vi "EOL Check Current Data.vi"(0 "Motor Type":T1, 5 "Motion Data":sgl[][](array[numeric]), 7 "Decibel data":dbl[](array[numeric]), 9 "Current Motion":T2=enum."Glass Slide Open", 11 "Audit Motion Data Cluster":T3={"Power Supply Voltage"=0.0, "Min Avg Current"=0.0, "Max Avg Current"=0.0, "Min Run Time"=0.0, "Max Run Time"=0.0, "Min Speed"=0.0, "Max Speed"=0.0, "AP Data % of Threshold"=0.0, "Travel Distance"=0.0, "AP Data Type"=enum."91/61", "Check Current"=FALSE, "Check Run Time"=FALSE, "Check Speed"=FALSE, "Express Motion?"=FALSE, "Check Sound Test"=FALSE, "Check Position?"=FALSE, "Collect AP Data"=FALSE, "Inital Position"=0, "End Position"=0, "Goto Posiition"=0, "Max max Current"=0.0, "Min max Current"=0.0, "Check max Current"=FALSE, "Check Sound"=FALSE, "Min Sound (dB)"=0.0, "Max Sound (dB)"=0.0, "SW Mode"=enum."Hard Switch", "LIN Msg"={"ID"=0, "Msg"=[], "LDF"="EX1H"}} {"LIN Msg"."Msg" format="%02x"; "LIN Msg"."ID" format="%02x"}, 12 "Error Table In":string[][](array[string])) -> (1 "max Current":dbl, 3 "Current Out":sgl[](graph), 4 "Pass? Out":bool, 6 "Run Time":dbl, 8 "Sound (dB)":dbl, 10 "Avg Current":dbl, 14 "Error Table Out":string[][](array[string]), 15 "Speed":dbl)   [LabVIEW 2018]
uses:
  05.UserVI's/type defs/17x Audit Motion Data Seq Control.ctl
  05.UserVI's/type defs/17x AP Data Type.ctl
  02.Type Def's/All Motions.ctl
  05.UserVI's/type defs/EOL Motor Type.ctl
  <vilib>/Analysis/baseanly.llb/Mean (DBL).vi
  <vilib>/Analysis/NI_AALBase.lvlib
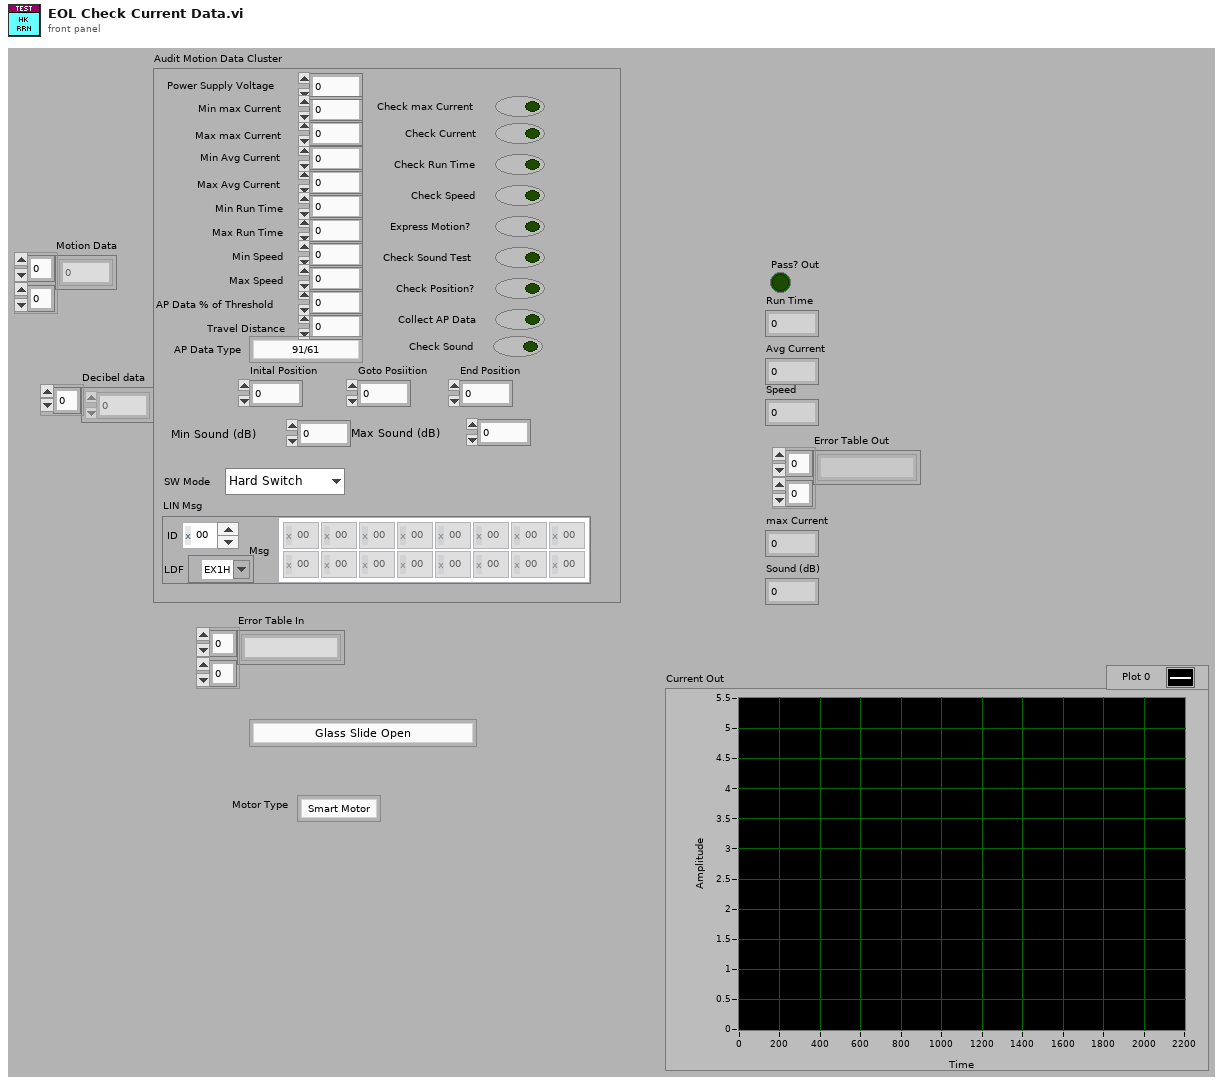
[diagram p1: front panel]
types:
  T1 = typedef "EOL Motor Type.ctl" = enum16{"Smart Motor", "Sensor Motor"}
  T2 = typedef "All Motions.ctl" = enum16{"Glass Teach", "Glass Slide Open", "Glass Slide Close", "Glass Vent Open", "Glass Vent Close", "Sunshade Teach", "Sunshade Open", "Sunshade Close", "Idle", "Sunshade Open 2", "Sunshade Close 2", "Glass Slide Open Sunshade Open", "Glass Slide Open Sunshade Close", "Glass Slide Close Sunshade Open", "Glass Slide Close Sunshade Close", "Glass Vent Open Sunshade Open", "Glass Vent Open Sunshade Close", "Glass Vent Close Sunshade Open", "Glass Vent Close Sunshade Close", "Express Glass Slide Open", "Express Glass Slide Close", "Express Glass Vent Open", "Express Glass Vent Close", "Express Sunshade Open", "Express Sunshade Close", "Express Sunshade Open 2", "Express Sunshade Close 2", "Express Glass Slide Open Sunshade Open", "Express Glass Slide Open Sunshade Close", "Express Glass Slide Close Sunshade Open", "Express Glass Slide Close Sunshade Close", "Express Glass Vent Open Sunshade Open", "Express Glass Vent Open Sunshade Close", "Express Glass Vent Close Sunshade Open", "Express Glass Vent Close Sunshade Close", "Goto Position Glass", "Goto Position Sunshade", "Sunshade Teach 2"}
  T3 = typedef "17x Audit Motion Data Seq Control.ctl" = cluster{"Power Supply Voltage":dbl, "Min Avg Current":dbl, "Max Avg Current":dbl, "Min Run Time":dbl, "Max Run Time":dbl, "Min Speed":dbl, "Max Speed":dbl, "AP Data % of Threshold":dbl, "Travel Distance":dbl, "AP Data Type":T4, "Check Current":bool, "Check Run Time":bool, "Check Speed":bool, "Express Motion?":bool, "Check Sound Test":bool, "Check Position?":bool, "Collect AP Data":bool, "Inital Position":u16, "End Position":u16, "Goto Posiition":u16, "Max max Current":dbl, "Min max Current":dbl, "Check max Current":bool, "Check Sound":bool, "Min Sound (dB)":dbl, "Max Sound (dB)":dbl, "SW Mode":enum16{"Hard Switch", "Uncond Frame"}, "LIN Msg":cluster{"ID":u8, "Msg":u8[][], "LDF":refnum<k21>}}
  T4 = typedef "17x AP Data Type.ctl" = enum16{"91/61", "92/62", "93/63", "67", "68", "6F", "71", "91 Msg", "92 Msg", "93 Msg", "94 Msg", "HiRain 91", "HiRain 92 Speed", "HiRain 92 HS", "HiRain 92", "HiRain 93", "SnT"}
  T5 = cluster{"Run Time":dbl, "Avg Current":dbl, "Speed":dbl, "Audit Motion Data Cluster":T3, "Error Table In":string[][], "Pass?":bool, "Current Motion":T2, "Motor Type":T1, "max Current":dbl, "Sound (dB)":dbl, "Decibel data":dbl[]}
  T6 = typedef "EOL Analog Input Control.ctl" = enum16{"SW PS  Volage", "Switch A", "Switch B", "Switch C", "Motor Voltage", "Motor Current", "ATS"}
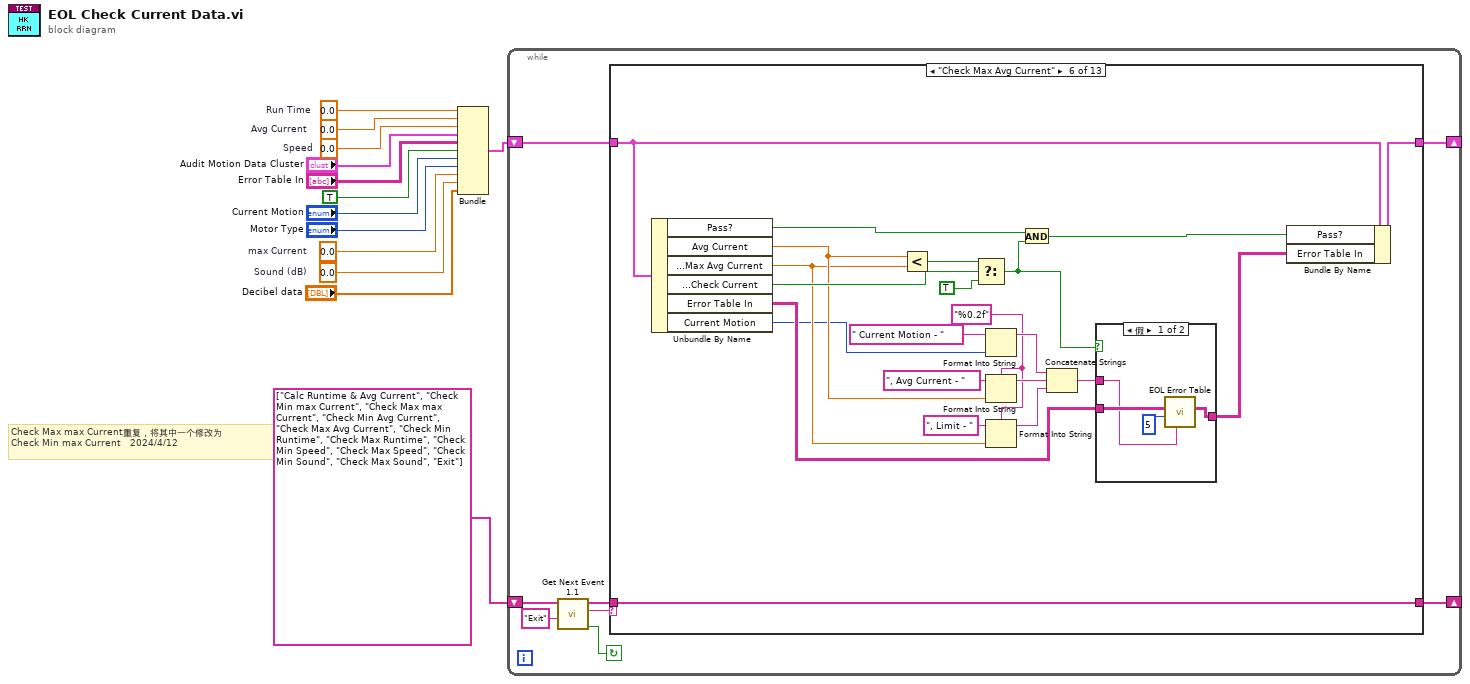
[diagram p0: block diagram]
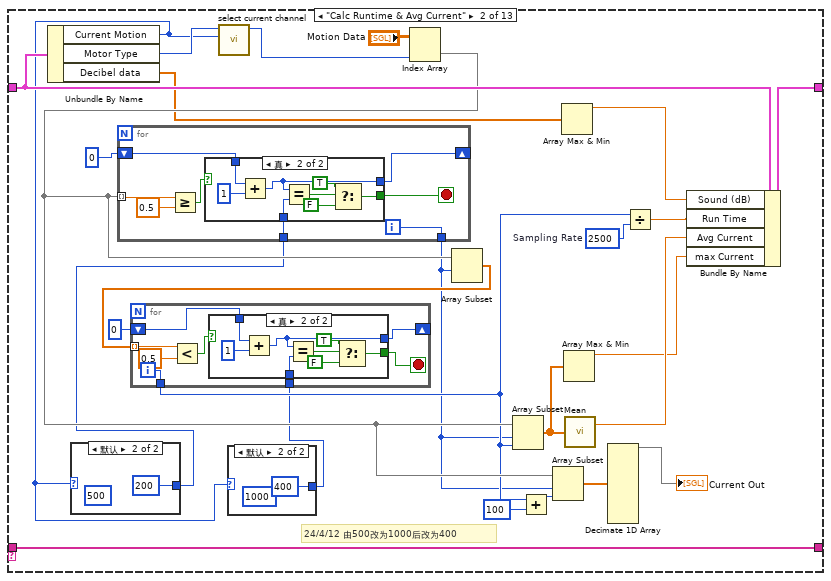
[diagram p3: hidden frame]
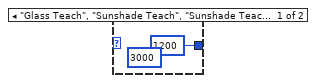
[diagram p4: hidden frame]
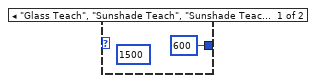
[diagram p5: hidden frame]
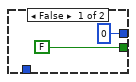
[diagram p6: hidden frame]
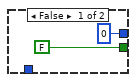
[diagram p7: hidden frame]
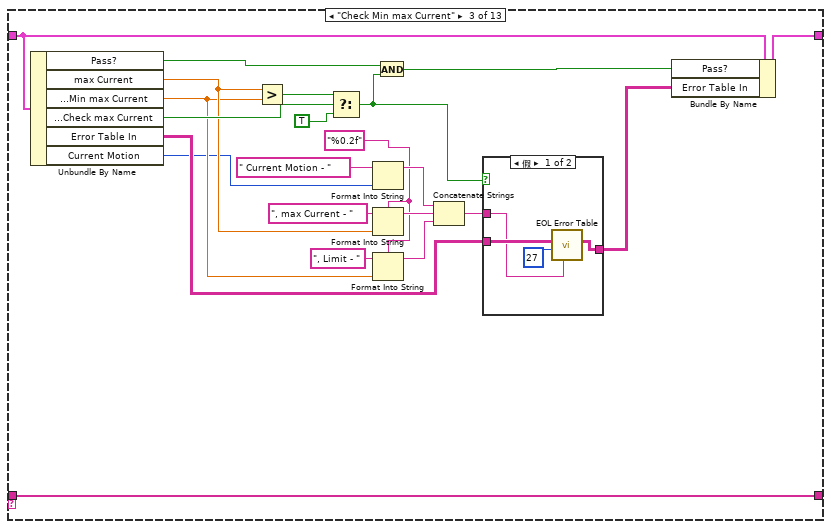
[diagram p8: hidden frame]
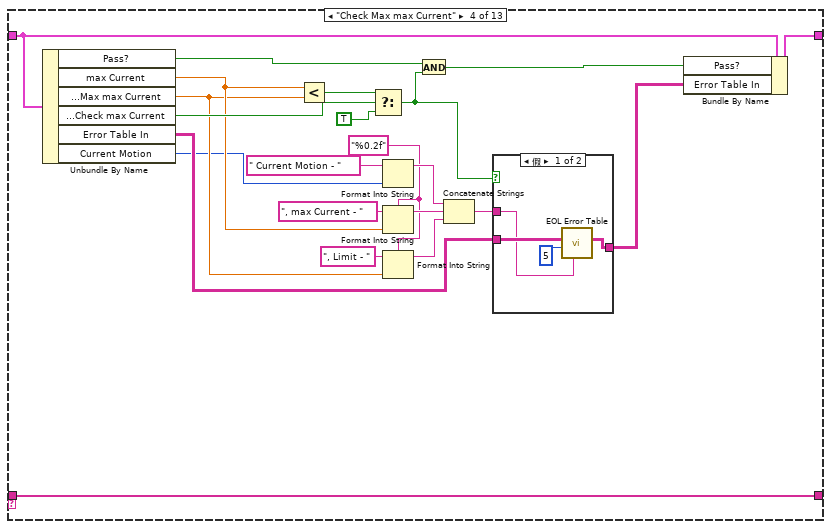
[diagram p10: hidden frame]
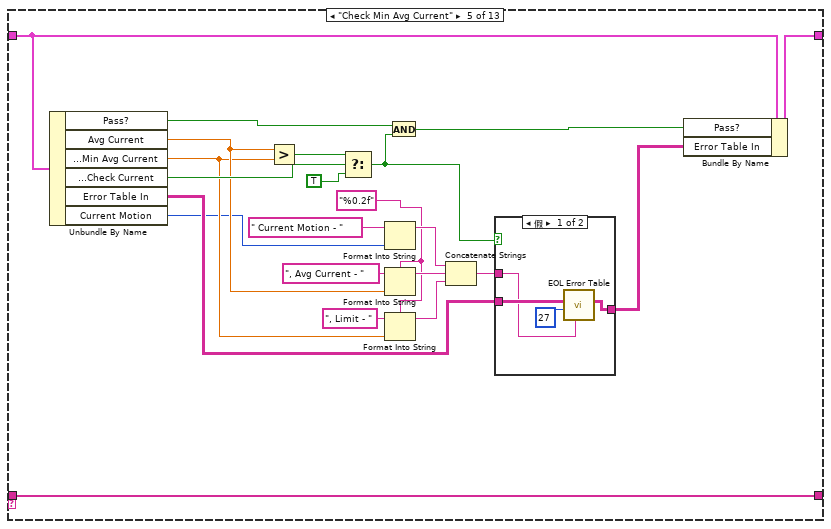
[diagram p12: hidden frame]
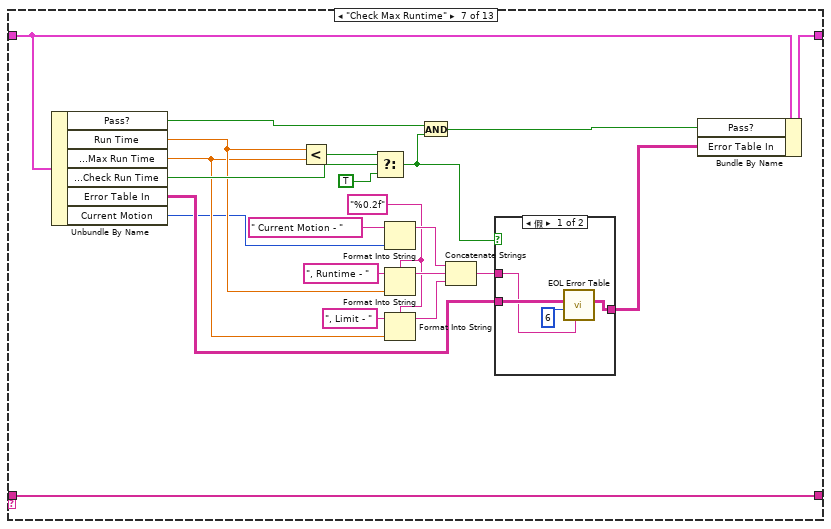
[diagram p15: hidden frame]
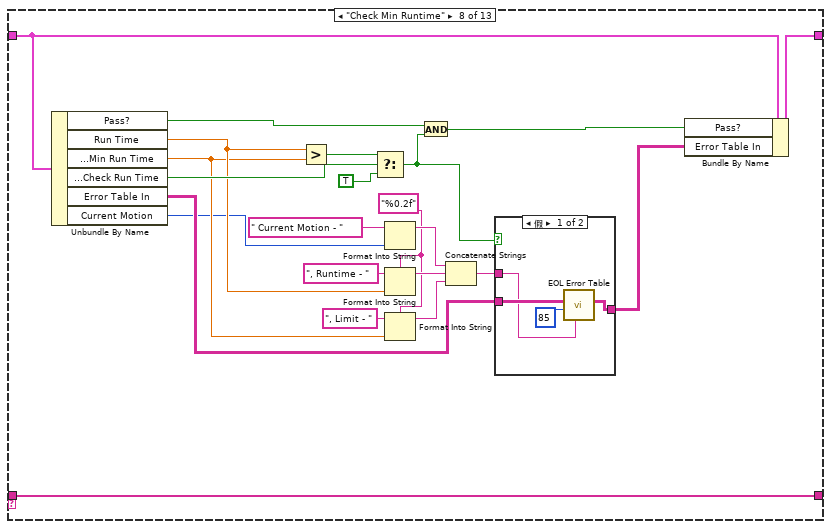
[diagram p17: hidden frame]
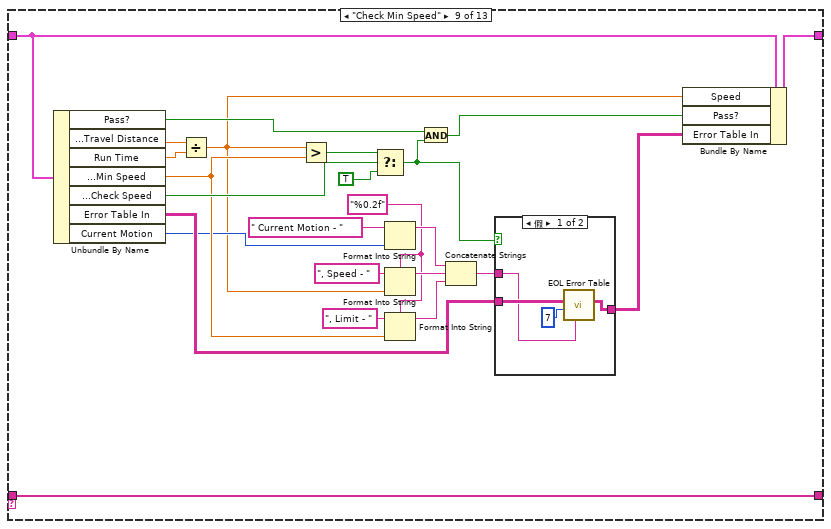
[diagram p19: hidden frame]
diagram:
  w2 = 0.0  # Sound (dB)
  w3 = 0.0  # max Current
  w5 = 0.0  # Speed
  w11 = 0.0  # Avg Current
  w12 = 0.0  # Run Time
  # "Check Max max Current重复，将其中一个修改为\nCheck Min max Current   2024/4/12"
  n1 = Bundle("Run Time"=w12, "Avg Current"=w11, "Speed"=w5, "Audit Motion Data Cluster"="Audit Motion Data Cluster", "Error Table In"="Error Table In", "Pass?"=TRUE, "Current Motion"="Current Motion", "Motor Type"="Motor Type", "max Current"=w3, "Sound (dB)"=w2, "Decibel data"="Decibel data") -> (w10:T5)  [unwired: 1 in]
  n2 = while {
    shift-right: [w19] -> _
    shift-left: string[] ["Calc Runtime & Avg Current", "Check Min max Current", "Check Max max Current", "Check Min Avg Current", "Check Max Avg Current", "Check Min Runtime", "Check Max Runtime", "Check Min Speed", "Check Max Speed", "Check Min Sound", "Check Max Sound", "Exit"] ("event queue out") -> [w18]
    shift-right: [w14] -> _
    shift-left: w10 -> [w15]
    stop <- w16 continue-if-true
    n3 = call "Get Next Event 1.1.vi"("Exit Event"="Exit", "event queue in"=w18) -> ("Condition (Exit:F)"=w16:bool, "next event"=w21:string, "event queue out"=w20:string[])  [unwired: 6 in, 1 out]
    n4 = case shown="\"Check Max Avg Current\"" w21 {
      tunnel: w20 -> [w23 w49 w90 w117 w165 w192 w219 w246 w275 w304 w311 w358 w372]
      tunnel: [w23 w49 w90 w117 w165 w192 w219 w246 w275 w304 w311 w358 w372] -> w19
      tunnel: w15 -> [w22 w40 w92 w119 w149 w176 w203 w230 w260 w289 w313 w338 w366]
      tunnel: [w22 w45 w91 w118 w145 w172 w199 w226 w253 w282 w312 w337 w366] -> w14
      frame "Error", Default {
      }
      frame "Calc Runtime & Avg Current" {
        w48 = 2500  # Sampling Rate
        # "24/4/12 由500改为1000后改为400"
        n5 = Unbundle By Name(w40) -> ("Current Motion"=w25:T2, "Motor Type"=w39:T1, "Decibel data"=w27:dbl[])
        n6 = case shown="默认" w25 {
          tunnel: [600 ("y") 200 ("y")] -> w26
          frame "Glass Teach", "Sunshade Teach", "Sunshade Teach 2" {
            (unwired) 1500 ("y")
          }
          frame Default {
            (unwired) 500 ("y")
          }
        }
        n7 = call "select current channel.vi"("Current Motion"=w25, "Motor Type"=w39) -> ("Analog channel"=w37:T6)  [unwired: 9 in]
        n8 = case shown="默认" w25 {
          tunnel: [1200 ("y") 400 ("y")] -> w24
          frame "Glass Teach", "Sunshade Teach", "Sunshade Teach 2" {
            (unwired) 3000 ("y")
          }
          frame Default {
            (unwired) 1000 ("y")
          }
        }
        n9 = Index Array(array="Motion Data", index (col)=w37) -> (element=w31:sgl[])  [unwired: 1 in]
        n10 = for {
          tunnel: w31 -> [w56] mode=indexing
          tunnel: [w61] -> w29
          shift-right: [w59] -> _
          shift-left: 0 -> [w60]
          tunnel: w26 -> [w54]
          i -> [w61]
          stop <- w58 stop-if-true
          n11 = Greater Or Equal?(x=w56, y=sgl 0.5) -> (x >= y?=w55:bool)
          n12 = case shown="真" w55 {
            tunnel: w60 -> [_ w71]
            tunnel: [0 w69] -> w59
            tunnel: [FALSE w65] -> w58
            tunnel: w54 -> [_ w64]
            frame False {
            }
            frame True {
              n13 = Add(x=w71, y=1) -> (x+y=w69:i32)
              n14 = Equal?(x=w69, y=w64) -> (x = y?=w68:bool)
              n15 = Select(t=TRUE, s=w68, f=FALSE) -> (s? t:f=w65:bool)
            }
          }
        }
        n16 = Array Subset(array=w31, index=w29) -> (w32:sgl[])  [unwired: 1 in]
        n17 = for {
          tunnel: w32 -> [w74] mode=indexing
          tunnel: [w79] -> w30
          shift-right: [w78] -> _
          shift-left: 0 -> [w77]
          tunnel: w24 -> [w72]
          i -> [w79]
          stop <- w76 stop-if-true
          n18 = Less?(x=w74, y=sgl 0.5) -> (x < y?=w73:bool)
          n19 = case shown="真" w73 {
            tunnel: w77 -> [_ w89]
            tunnel: [0 w87] -> w78
            tunnel: [FALSE w83] -> w76
            tunnel: w72 -> [_ w82]
            frame False {
            }
            frame True {
              n20 = Add(x=w89, y=1) -> (x+y=w87:i32)
              n21 = Equal?(x=w87, y=w82) -> (x = y?=w86:bool)
              n22 = Select(t=TRUE, s=w86, f=FALSE) -> (s? t:f=w83:bool)
            }
          }
        }
        n23 = Array Subset(array=w31, index=w29, length=w30) -> (w36:sgl[])
        n24 = Add(x=w30, y=100) -> (x+y=w44:i32)
        n25 = Array Subset(array=w31, index=w29, length=w44) -> (w42:sgl[])
        n26 = Array Max & Min(array=w27) -> (max value=w28:dbl)  [unwired: 3 out]
        n27 = Array Max & Min(array=w36) -> (max value=w35:sgl)  [unwired: 3 out]
        n28 = call-poly <vilib>:"Mean.vi"("X"=w36) -> ("mean"=w46:dbl)  [unwired: 1 out]
        n29 = Decimate 1D Array(w42) -> (→"Current Out":sgl[])  [unwired: 9 out]
        n30 = Divide(x=w30, y=w48) -> (x/y=w47:dbl)
        n31 = Bundle By Name(cluster=w40, "Sound (dB)"=w28, "Run Time"=w47, "Avg Current"=w46, "max Current"=w35) -> (w45:T5)
      }
      frame "Check Min max Current" {
        w93 = "%0.2f" ("format string")
        n32 = Unbundle By Name(w92) -> ("Pass?"=w97:bool, "max Current"=w101:dbl, "Audit Motion Data Cluster.Min max Current"=w100:dbl, "Audit Motion Data Cluster.Check max Current"=w110:bool, "Error Table In"=w99:string[][], "Current Motion"=w94:T2)
        n33 = Greater?(x=w101, y=w100) -> (0:w109:bool)
        n34 = Select(t=w109, s=w110, f=TRUE) -> (s? t:f=w98:bool)
        n35 = Format Into String(initial string=" Current Motion - ", w94) -> (resulting string=w105:string)  [unwired: 2 in, 1 out]
        n36 = Format Into String(format string=w93, initial string=", max Current - ", w101) -> (resulting string=w106:string)  [unwired: 1 in, 1 out]
        n37 = Format Into String(format string=w93, initial string=", Limit - ", w100) -> (resulting string=w107:string)  [unwired: 1 in, 1 out]
        n38 = And(x=w97, y=w98) -> (x .and. y?=w95:bool)
        n39 = Concatenate Strings(w105, w106, w107) -> (w108:string)
        n40 = case shown="假" w98 {
          tunnel: w99 -> [w115 w116]
          tunnel: w108 -> [w113 _]
          tunnel: [w112 w116] -> w96
          frame False {
            n41 = call "EOL Error Table.vi"("Error Description"=w113, "Error No."=u16 27, "Error Table In"=w115) -> ("Error Table Out"=w112:string[][])  [unwired: 7 in, 1 out]
          }
          frame True {
          }
        }
        n42 = Bundle By Name(cluster=w92, "Pass?"=w95, "Error Table In"=w96) -> (w91:T5)
      }
      frame "Check Max max Current" {
        w120 = "%0.2f" ("format string")
        n43 = Unbundle By Name(w119) -> ("Pass?"=w124:bool, "max Current"=w128:dbl, "Audit Motion Data Cluster.Max max Current"=w127:dbl, "Audit Motion Data Cluster.Check max Current"=w137:bool, "Error Table In"=w126:string[][], "Current Motion"=w121:T2)
        n44 = Less?(x=w128, y=w127) -> (x < y?=w136:bool)
        n45 = Select(t=w136, s=w137, f=TRUE) -> (s? t:f=w125:bool)
        n46 = Format Into String(initial string=" Current Motion - ", w121) -> (resulting string=w132:string)  [unwired: 2 in, 1 out]
        n47 = Format Into String(format string=w120, initial string=", max Current - ", w128) -> (resulting string=w133:string)  [unwired: 1 in, 1 out]
        n48 = Format Into String(format string=w120, initial string=", Limit - ", w127) -> (resulting string=w134:string)  [unwired: 1 in, 1 out]
        n49 = And(x=w124, y=w125) -> (x .and. y?=w122:bool)
        n50 = Concatenate Strings(w132, w133, w134) -> (w135:string)
        n51 = case shown="假" w125 {
          tunnel: w126 -> [w142 w143]
          tunnel: w135 -> [w141 _]
          tunnel: [w139 w143] -> w123
          frame False {
            n52 = call "EOL Error Table.vi"("Error Description"=w141, "Error No."=u16 5, "Error Table In"=w142) -> ("Error Table Out"=w139:string[][])  [unwired: 7 in, 1 out]
          }
          frame True {
          }
        }
        n53 = Bundle By Name(cluster=w119, "Pass?"=w122, "Error Table In"=w123) -> (w118:T5)
      }
      frame "Check Min Avg Current" {
        w144 = "%0.2f" ("format string")
        n54 = Unbundle By Name(w149) -> ("Pass?"=w150:bool, "Avg Current"=w154:dbl, "Audit Motion Data Cluster.Min Avg Current"=w153:dbl, "Audit Motion Data Cluster.Check Current"=w163:bool, "Error Table In"=w152:string[][], "Current Motion"=w146:T2)
        n55 = Greater?(x=w154, y=w153) -> (0:w162:bool)
        n56 = Select(t=w162, s=w163, f=TRUE) -> (s? t:f=w151:bool)
        n57 = Format Into String(initial string=" Current Motion - ", w146) -> (resulting string=w158:string)  [unwired: 2 in, 1 out]
        n58 = Format Into String(format string=w144, initial string=", Avg Current - ", w154) -> (resulting string=w159:string)  [unwired: 1 in, 1 out]
        n59 = Format Into String(format string=w144, initial string=", Limit - ", w153) -> (resulting string=w160:string)  [unwired: 1 in, 1 out]
        n60 = And(x=w150, y=w151) -> (x .and. y?=w147:bool)
        n61 = Concatenate Strings(w158, w159, w160) -> (w161:string)
        n62 = case shown="假" w151 {
          tunnel: w152 -> [w169 w170]
          tunnel: w161 -> [w167 _]
          tunnel: [w166 w170] -> w148
          frame False {
            n63 = call "EOL Error Table.vi"("Error Description"=w167, "Error No."=u16 27, "Error Table In"=w169) -> ("Error Table Out"=w166:string[][])  [unwired: 7 in, 1 out]
          }
          frame True {
          }
        }
        n64 = Bundle By Name(cluster=w149, "Pass?"=w147, "Error Table In"=w148) -> (w145:T5)
      }
      frame "Check Max Avg Current" {
        w171 = "%0.2f" ("format string")
        n65 = Unbundle By Name(w176) -> ("Pass?"=w177:bool, "Avg Current"=w181:dbl, "Audit Motion Data Cluster.Max Avg Current"=w180:dbl, "Audit Motion Data Cluster.Check Current"=w190:bool, "Error Table In"=w179:string[][], "Current Motion"=w173:T2)
        n66 = Less?(x=w181, y=w180) -> (x < y?=w189:bool)
        n67 = Select(t=w189, s=w190, f=TRUE) -> (s? t:f=w178:bool)
        n68 = Format Into String(initial string=" Current Motion - ", w173) -> (resulting string=w185:string)  [unwired: 2 in, 1 out]
        n69 = Format Into String(format string=w171, initial string=", Avg Current - ", w181) -> (resulting string=w186:string)  [unwired: 1 in, 1 out]
        n70 = Format Into String(format string=w171, initial string=", Limit - ", w180) -> (resulting string=w187:string)  [unwired: 1 in, 1 out]
        n71 = And(x=w177, y=w178) -> (x .and. y?=w174:bool)
        n72 = Concatenate Strings(w185, w186, w187) -> (w188:string)
        n73 = case shown="假" w178 {
          tunnel: w179 -> [w196 w197]
          tunnel: w188 -> [w195 _]
          tunnel: [w193 w197] -> w175
          frame False {
            n74 = call "EOL Error Table.vi"("Error Description"=w195, "Error No."=u16 5, "Error Table In"=w196) -> ("Error Table Out"=w193:string[][])  [unwired: 7 in, 1 out]
          }
          frame True {
          }
        }
        n75 = Bundle By Name(cluster=w176, "Pass?"=w174, "Error Table In"=w175) -> (w172:T5)
      }
      frame "Check Max Runtime" {
        w198 = "%0.2f" ("format string")
        n76 = Unbundle By Name(w203) -> ("Pass?"=w204:bool, "Run Time"=w208:dbl, "Audit Motion Data Cluster.Max Run Time"=w207:dbl, "Audit Motion Data Cluster.Check Run Time"=w217:bool, "Error Table In"=w206:string[][], "Current Motion"=w200:T2)
        n77 = Less?(x=w208, y=w207) -> (x < y?=w216:bool)
        n78 = Select(t=w216, s=w217, f=TRUE) -> (s? t:f=w205:bool)
        n79 = Format Into String(initial string=" Current Motion - ", w200) -> (resulting string=w212:string)  [unwired: 2 in, 1 out]
        n80 = Format Into String(format string=w198, initial string=", Runtime - ", w208) -> (resulting string=w213:string)  [unwired: 1 in, 1 out]
        n81 = Format Into String(format string=w198, initial string=", Limit - ", w207) -> (resulting string=w214:string)  [unwired: 1 in, 1 out]
        n82 = And(x=w204, y=w205) -> (x .and. y?=w201:bool)
        n83 = Concatenate Strings(w212, w213, w214) -> (w215:string)
        n84 = case shown="假" w205 {
          tunnel: w206 -> [w223 w224]
          tunnel: w215 -> [w221 _]
          tunnel: [w220 w224] -> w202
          frame False {
            n85 = call "EOL Error Table.vi"("Error Description"=w221, "Error No."=u16 6, "Error Table In"=w223) -> ("Error Table Out"=w220:string[][])  [unwired: 7 in, 1 out]
          }
          frame True {
          }
        }
        n86 = Bundle By Name(cluster=w203, "Pass?"=w201, "Error Table In"=w202) -> (w199:T5)
      }
      frame "Check Min Runtime" {
        w225 = "%0.2f" ("format string")
        n87 = Unbundle By Name(w230) -> ("Pass?"=w231:bool, "Run Time"=w235:dbl, "Audit Motion Data Cluster.Min Run Time"=w234:dbl, "Audit Motion Data Cluster.Check Run Time"=w244:bool, "Error Table In"=w233:string[][], "Current Motion"=w227:T2)
        n88 = Greater?(x=w235, y=w234) -> (0:w243:bool)
        n89 = Select(t=w243, s=w244, f=TRUE) -> (s? t:f=w232:bool)
        n90 = Format Into String(initial string=" Current Motion - ", w227) -> (resulting string=w239:string)  [unwired: 2 in, 1 out]
        n91 = Format Into String(format string=w225, initial string=", Runtime - ", w235) -> (resulting string=w240:string)  [unwired: 1 in, 1 out]
        n92 = Format Into String(format string=w225, initial string=", Limit - ", w234) -> (resulting string=w241:string)  [unwired: 1 in, 1 out]
        n93 = And(x=w231, y=w232) -> (x .and. y?=w228:bool)
        n94 = Concatenate Strings(w239, w240, w241) -> (w242:string)
        n95 = case shown="假" w232 {
          tunnel: w233 -> [w250 w251]
          tunnel: w242 -> [w248 _]
          tunnel: [w247 w251] -> w229
          frame False {
            n96 = call "EOL Error Table.vi"("Error Description"=w248, "Error No."=u16 85, "Error Table In"=w250) -> ("Error Table Out"=w247:string[][])  [unwired: 7 in, 1 out]
          }
          frame True {
          }
        }
        n97 = Bundle By Name(cluster=w230, "Pass?"=w228, "Error Table In"=w229) -> (w226:T5)
      }
      frame "Check Min Speed" {
        w252 = "%0.2f" ("format string")
        n98 = Unbundle By Name(w260) -> ("Pass?"=w261:bool, "Audit Motion Data Cluster.Travel Distance"=w256:dbl, "Run Time"=w255:dbl, "Audit Motion Data Cluster.Min Speed"=w264:dbl, "Audit Motion Data Cluster.Check Speed"=w273:bool, "Error Table In"=w263:string[][], "Current Motion"=w257:T2)
        n99 = Divide(x=w256, y=w255) -> (x/y=w254:dbl)
        n100 = Greater?(x=w254, y=w264) -> (0:w272:bool)
        n101 = Select(t=w272, s=w273, f=TRUE) -> (s? t:f=w262:bool)
        n102 = Format Into String(initial string=" Current Motion - ", w257) -> (resulting string=w268:string)  [unwired: 2 in, 1 out]
        n103 = Format Into String(format string=w252, initial string=", Speed - ", w254) -> (resulting string=w269:string)  [unwired: 1 in, 1 out]
        n104 = Format Into String(format string=w252, initial string=", Limit - ", w264) -> (resulting string=w270:string)  [unwired: 1 in, 1 out]
        n105 = And(x=w261, y=w262) -> (x .and. y?=w258:bool)
        n106 = Concatenate Strings(w268, w269, w270) -> (w271:string)
        n107 = case shown="假" w262 {
          tunnel: w263 -> [w279 w280]
          tunnel: w271 -> [w277 _]
          tunnel: [w276 w280] -> w259
          frame False {
            n108 = call "EOL Error Table.vi"("Error Description"=w277, "Error No."=u16 7, "Error Table In"=w279) -> ("Error Table Out"=w276:string[][])  [unwired: 7 in, 1 out]
          }
          frame True {
          }
        }
        n109 = Bundle By Name(cluster=w260, "Speed"=w254, "Pass?"=w258, "Error Table In"=w259) -> (w253:T5)
      }
      frame "Check Max Speed" {
        w281 = "%0.2f" ("format string")
        n110 = Unbundle By Name(w289) -> ("Pass?"=w290:bool, "Audit Motion Data Cluster.Travel Distance"=w285:dbl, "Run Time"=w284:dbl, "Audit Motion Data Cluster.Max Speed"=w293:dbl, "Audit Motion Data Cluster.Check Speed"=w302:bool, "Error Table In"=w292:string[][], "Current Motion"=w286:T2)
        n111 = Divide(x=w285, y=w284) -> (x/y=w283:dbl)
        n112 = Less?(x=w283, y=w293) -> (x < y?=w301:bool)
        n113 = Select(t=w301, s=w302, f=TRUE) -> (s? t:f=w291:bool)
        n114 = Format Into String(initial string=" Current Motion - ", w286) -> (resulting string=w297:string)  [unwired: 2 in, 1 out]
        n115 = Format Into String(format string=w281, initial string=", Speed - ", w283) -> (resulting string=w298:string)  [unwired: 1 in, 1 out]
        n116 = Format Into String(format string=w281, initial string=", Limit - ", w293) -> (resulting string=w299:string)  [unwired: 1 in, 1 out]
        n117 = And(x=w290, y=w291) -> (x .and. y?=w287:bool)
        n118 = Concatenate Strings(w297, w298, w299) -> (w300:string)
        n119 = case shown="假" w291 {
          tunnel: w292 -> [w308 w309]
          tunnel: w300 -> [w306 _]
          tunnel: [w305 w309] -> w288
          frame False {
            n120 = call "EOL Error Table.vi"("Error Description"=w306, "Error No."=u16 84, "Error Table In"=w308) -> ("Error Table Out"=w305:string[][])  [unwired: 7 in, 1 out]
          }
          frame True {
          }
        }
        n121 = Bundle By Name(cluster=w289, "Speed"=w283, "Pass?"=w287, "Error Table In"=w288) -> (w282:T5)
      }
      frame "Check Min Sound" {
        w314 = "%0.2f" ("format string")
        n122 = Unbundle By Name(w313) -> ("Pass?"=w318:bool, "Sound (dB)"=w310:dbl, "Audit Motion Data Cluster.Min Sound (dB)"=w321:dbl, "Audit Motion Data Cluster.Check Sound"=w330:bool, "Error Table In"=w320:string[][], "Current Motion"=w315:T2)
        n123 = Greater Or Equal?(x=w310, y=w321) -> (x >= y?=w329:bool)
        n124 = Select(t=w329, s=w330, f=TRUE) -> (s? t:f=w319:bool)
        n125 = Format Into String(initial string=" Current Motion - ", w315) -> (resulting string=w325:string)  [unwired: 2 in, 1 out]
        n126 = Format Into String(format string=w314, initial string=", Sound - ", w310) -> (resulting string=w326:string)  [unwired: 1 in, 1 out]
        n127 = Format Into String(format string=w314, initial string=", Limit - ", w321) -> (resulting string=w327:string)  [unwired: 1 in, 1 out]
        n128 = And(x=w318, y=w319) -> (x .and. y?=w316:bool)
        n129 = Concatenate Strings(w325, w326, w327) -> (w328:string)
        n130 = case shown="假" w319 {
          tunnel: w320 -> [w335 w336]
          tunnel: w328 -> [w333 _]
          tunnel: [w332 w336] -> w317
          frame False {
            n131 = call "EOL Error Table.vi"("Error Description"=w333, "Error No."=u16 210, "Error Table In"=w335) -> ("Error Table Out"=w332:string[][])  [unwired: 7 in, 1 out]
          }
          frame True {
          }
        }
        n132 = Bundle By Name(cluster=w313, "Sound (dB)"=w310, "Pass?"=w316, "Error Table In"=w317) -> (w312:T5)
      }
      frame "Check Max Sound" {
        w340 = "%0.2f" ("format string")
        n133 = Unbundle By Name(w338) -> ("Pass?"=w344:bool, "Sound (dB)"=w339:dbl, "Audit Motion Data Cluster.Max Sound (dB)"=w347:dbl, "Audit Motion Data Cluster.Check Sound"=w356:bool, "Error Table In"=w346:string[][], "Current Motion"=w341:T2)
        n134 = Less Or Equal?(x=w339, y=w347) -> (x <= y?=w355:bool)
        n135 = Select(t=w355, s=w356, f=TRUE) -> (s? t:f=w345:bool)
        n136 = Format Into String(initial string=" Current Motion - ", w341) -> (resulting string=w351:string)  [unwired: 2 in, 1 out]
        n137 = Format Into String(format string=w340, initial string=", Sound - ", w339) -> (resulting string=w352:string)  [unwired: 1 in, 1 out]
        n138 = Format Into String(format string=w340, initial string=", Limit - ", w347) -> (resulting string=w353:string)  [unwired: 1 in, 1 out]
        n139 = And(x=w344, y=w345) -> (x .and. y?=w342:bool)
        n140 = Concatenate Strings(w351, w352, w353) -> (w354:string)
        n141 = case shown="假" w345 {
          tunnel: w346 -> [w362 w363]
          tunnel: w354 -> [w360 _]
          tunnel: [w359 w363] -> w343
          frame False {
            n142 = call "EOL Error Table.vi"("Error Description"=w360, "Error No."=u16 211, "Error Table In"=w362) -> ("Error Table Out"=w359:string[][])  [unwired: 7 in, 1 out]
          }
          frame True {
          }
        }
        n143 = Bundle By Name(cluster=w338, "Sound (dB)"=w339, "Pass?"=w342, "Error Table In"=w343) -> (w337:T5)
      }
      frame "Exit" {
        n144 = Unbundle By Name(w366) -> ("max Current"=→"max Current":dbl, "Run Time"=→"Run Time":dbl, "Avg Current"=→"Avg Current":dbl, "Speed"=→"Speed":dbl, "Pass?"=→"Pass? Out":bool, "Error Table In"=→"Error Table Out":string[][], "Sound (dB)"=→"Sound (dB)":dbl)
      }
    }
  }
